vi "MDAQ_Parse_BINSpectrum.vi"(8 "error in":errorcluster, 9 "?":T1 {"GATESTOP" format="%04x"; "GATESTRT" format="%04x"; "AMPLITUDE" format="%04x"; "M_CYCLES" format="%04x"; "N_CYCLES" format="%04x"; "STEP" format="%04x"; "BASE" format="%04x"; "CHAN" format="%04x"}, 10 "input buffer":string) -> (0 "error out":errorcluster, 1 "output cluster":T1 {"GATESTOP" format="%04x"; "GATESTRT" format="%04x"; "AMPLITUDE" format="%04x"; "M_CYCLES" format="%04x"; "N_CYCLES" format="%04x"; "STEP" format="%04x"; "BASE" format="%04x"; "CHAN" format="%04x"}, 2 "Array":u32[](array[numeric]))   [LabVIEW 2021]
uses:
  Status_Cluster.ctl
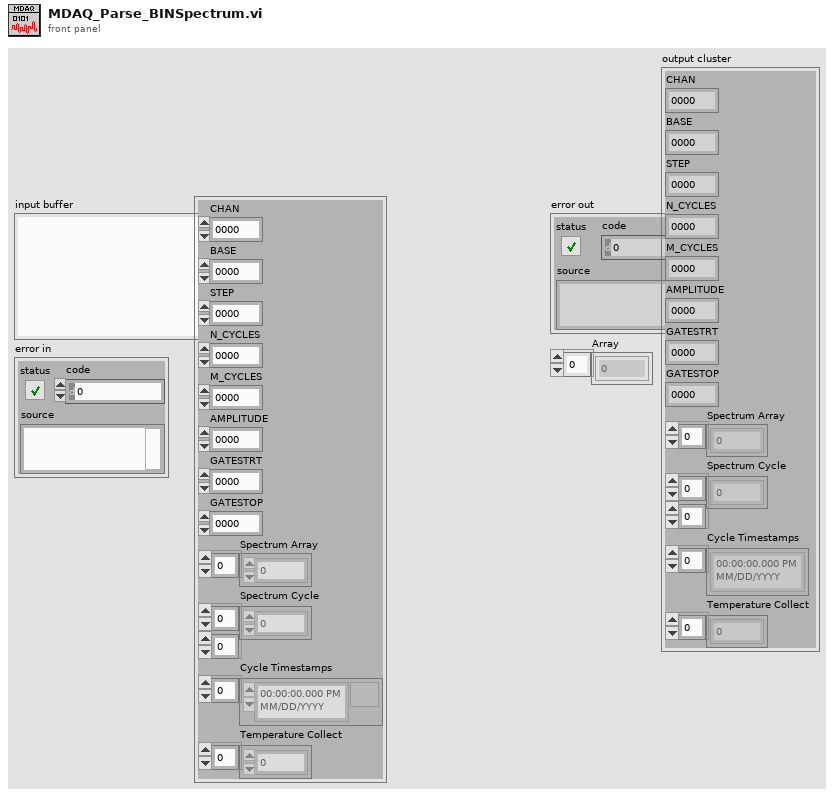
[diagram p1: front panel]
types:
  T1 = typedef "Status_Cluster.ctl" = cluster{"CHAN":u32, "BASE":u32, "STEP":u32, "N_CYCLES":u32, "M_CYCLES":u32, "AMPLITUDE":u32, "GATESTRT":u32, "GATESTOP":u32, "Spectrum Array":u32[], "Spectrum Cycle":u32[][], "Cycle Timestamps":timestamp[], "Temperature Collect":dbl[]}
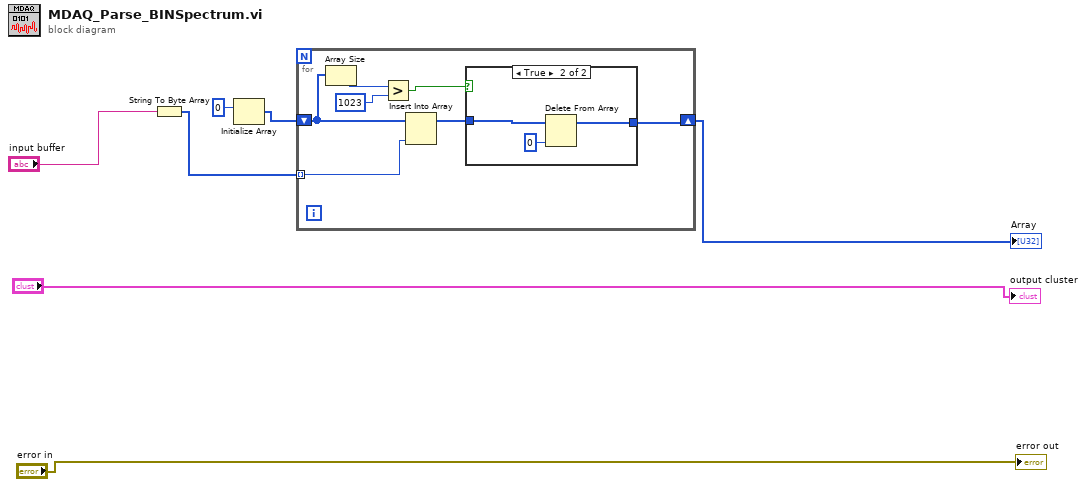
[diagram p0: block diagram]
diagram:
  n1 = String To Byte Array(string="input buffer") -> (unsigned byte array=w4:u8[])
  n2 = Initialize Array(0 ("element")) -> (w3:i32[])  [unwired: 1 in]
  n3 = for {
    tunnel: w4 -> [w9] mode=indexing
    shift-right: [w8] -> w1
    shift-left: w3 -> [w13]
    n4 = Array Size(array=w13) -> (size(s)=w12:i32)
    n5 = Greater?(x=w12, y=1023) -> (0:w10:bool)
    n6 = Insert Into Array(array=w13, new element=w9) -> (w14:i32[])  [unwired: 1 in]
    n7 = case shown="True" w10 {
      tunnel: w14 -> [w15 w18]
      tunnel: [w15 w16] -> w8
      frame False {
      }
      frame True {
        n8 = Delete From Array(array=w18, index=0) -> (array with subset deleted=w16:i32[])  [unwired: 1 in, 1 out]
      }
    }
  }
  "Array" <- w1
  "error out" <- "error in"
  "output cluster" <- "?"
